vi "Fetch Waveform Measurement In Memory.vi"(6 "Measurement Number (0: Measurement 1)":i32(ring) items=["Measurement 1", "Measurement 2", "Measurement 3", "Measurement 4"], 7 "Destination Channel (1: Channel 2)":u16(ring)=1 items=["Channel 1", "Channel 2", "Channel 3", "Channel 4", "Math", "D0", "D1", "D2", "D3", "D4", "D5", "D6", "D7", "D8", "D9", "D10", "D11", "D12", "D13", "D14", "D15", "Reference 1", "Reference 2", "Reference 3", "Reference 4", "Amplitude", "Frequency", "Phase"], 8 "error in (no error)":errorcluster, 9 "Measurement Function (21: Period)":i32(ring)=21 items=["Amplitude", "Area", "Burst Width", "Cycle Area", "Voltage Mean (cycle)", "Voltage RMS (cycle)", "Delay", "Fall Time", "Frequency", "Voltage High", "Voltage Low", "Voltage Max", "Voltage Mean", "Voltage Min", "Negative Duty Cycle", "Negative Edges Count", "Negative Overshoot", "Negative Pulses Count", "Negative Pulse Width", "Positive Duty Cycle", "Positive Edges Count", "Period", "Phase", "Vpp", "Positive Overshoot", "Positive Pulses Count", "Positive Pulse Width", "Rise Time", "Voltage RMS"], 10 "Channel (0: Channel 1)":u16(ring) items=["Channel 1", "Channel 2", "Channel 3", "Channel 4", "Math", "D0", "D1", "D2", "D3", "D4", "D5", "D6", "D7", "D8", "D9", "D10", "D11", "D12", "D13", "D14", "D15", "Reference 1", "Reference 2", "Reference 3", "Reference 4", "Amplitude", "Frequency", "Phase"], 11 "VISA resource name":refnum<visa-resource-name>) -> (0 "error out":errorcluster, 2 "Measurement Value":dbl, 3 "VISA resource name out":refnum<visa-resource-name>)   [LabVIEW 2009, in "Tektronix DPO MSO 2000 4000 Series.lvlib"]
doc: "This VI fetches the displayed measurement value which is specified by the <B>Measurement Number</B>. \n\nFirstly, initiates an acquisition on the channel that you specify in the <B>Channel</B> control. After the acquisition completes, the Fetch Displayed Waveform Measurement VI performs displayed waveform measurement on the channel you specify and returns a measurement value. You can specify a measurement type, such as rise time, frequency, and voltage peak-to-peak, with this VI. Use the Fetch Displayed Waveform Measurement VI separately for any other waveform measurement on a channel without initiating another acquisition.\n\n<B>Notes:</B>\n\nThe <B>Fetch Waveform Measurement</B> VI returns the immediate measurement (which is what is typically done) while this VI returns the specified displayed measurement."
uses:
  <instrlib>/Tektronix DPO MSO 2000 4000 Series/Tektronix DPO MSO 2000 4000 Series.lvlib
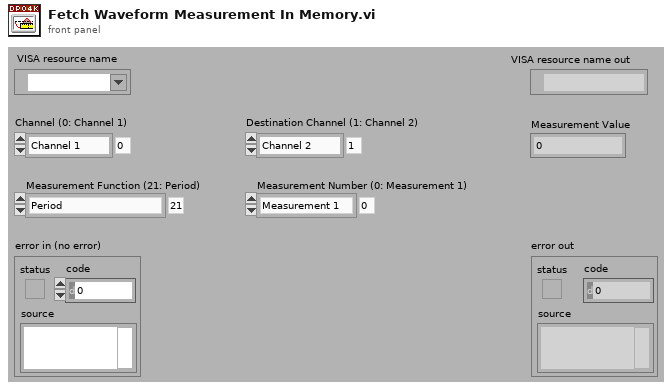
[diagram p1: front panel]
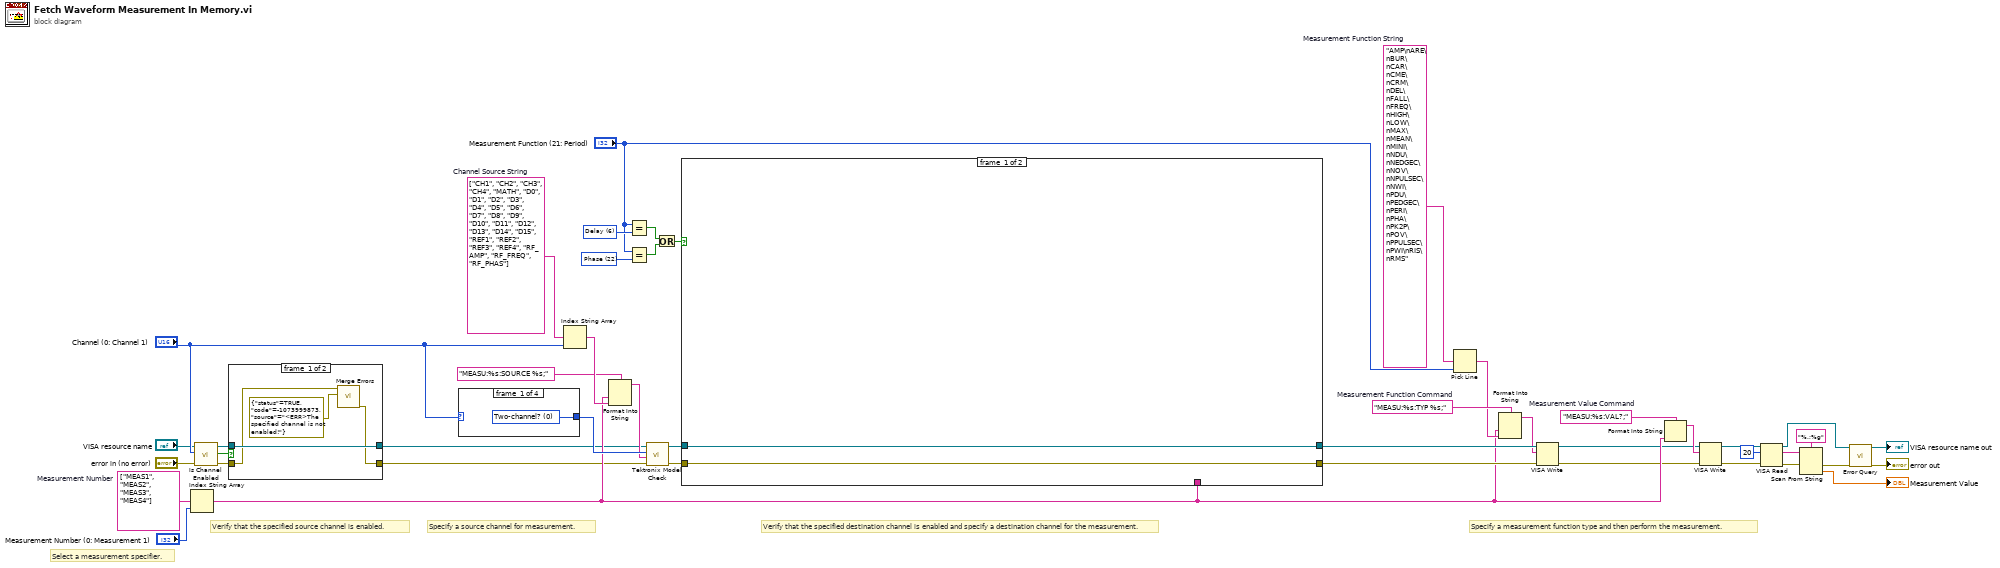
[diagram p0: block diagram]
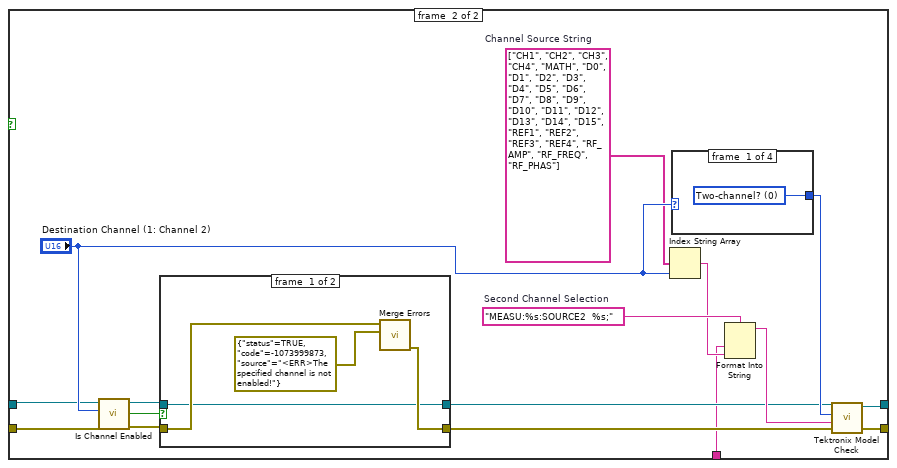
[diagram p2: hidden frame]
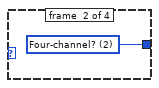
[diagram p3: hidden frame]
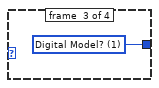
[diagram p4: hidden frame]
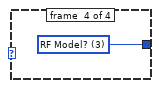
[diagram p5: hidden frame]
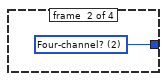
[diagram p7: hidden frame]
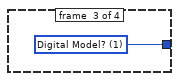
[diagram p8: hidden frame]
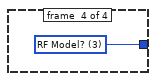
[diagram p9: hidden frame]
diagram:
  w11 = string[] ["MEAS1", "MEAS2", "MEAS3", "MEAS4"]  # Measurement Number
  w13 = "MEASU:%s:VAL?;"  # Measurement Value Command
  w28 = 22 items=["Amplitude", "Area", "Burst Width", "Cycle Area", "Voltage Mean (cycle)", "Voltage RMS (cycle)", "Delay", "Fall Time", "Frequency", "Voltage High", "Voltage Low", "Voltage Max", "Voltage Mean", "Voltage Min", "Negative Duty Cycle", "Negative Edges Count", "Negative Overshoot", "Negative Pulses Count", "Negative Pulse Width", "Positive Duty Cycle", "Positive Edges Count", "Period", "Phase", "Vpp", "Positive Overshoot", "Positive Pulses Count", "Positive Pulse Width", "Rise Time", "Voltage RMS"] ("Measurement Function (21: Period)")
  w29 = 6 items=["Amplitude", "Area", "Burst Width", "Cycle Area", "Voltage Mean (cycle)", "Voltage RMS (cycle)", "Delay", "Fall Time", "Frequency", "Voltage High", "Voltage Low", "Voltage Max", "Voltage Mean", "Voltage Min", "Negative Duty Cycle", "Negative Edges Count", "Negative Overshoot", "Negative Pulses Count", "Negative Pulse Width", "Positive Duty Cycle", "Positive Edges Count", "Period", "Phase", "Vpp", "Positive Overshoot", "Positive Pulses Count", "Positive Pulse Width", "Rise Time", "Voltage RMS"] ("Measurement Function (21: Period)")
  w37 = string[] ["CH1", "CH2", "CH3", "CH4", "MATH", "D0", "D1", "D2", "D3", "D4", "D5", "D6", "D7", "D8", "D9", "D10", "D11", "D12", "D13", "D14", "D15", "REF1", "REF2", "REF3", "REF4", "RF_AMP", "RF_FREQ", "RF_PHAS"]  # Channel Source String
  w44 = "MEASU:%s:TYP %s;"  # Measurement Function Command
  w45 = "AMP\nARE\nBUR\nCAR\nCME\nCRM\nDEL\nFALL\nFREQ\nHIGH\nLOW\nMAX\nMEAN\nMINI\nNDU\nNEDGEC\nNOV\nNPULSEC\nNWI\nPDU\nPEDGEC\nPERI\nPHA\nPK2P\nPOV\nPPULSEC\nPWI\nRIS\nRMS"  # Measurement Function String
  # "Select a measurement specifier."
  # "Specify a measurement function type and then perform the measurement."
  # "Specify a source channel for measurement."
  # "Verify that the specified destination channel is enabled and specify a destination channel for the measurement."
  # "Verify that the specified source channel is enabled."
  n1 = Index String Array(1:"Measurement Number (0: Measurement 1)", 2:w11) -> (0:w9:string)  [unwired: 1 in]
  n2 = call <instrlib>:"Is Channel Enabled.vi"("error in (no error)"="error in (no error)", "Channel (0: Channel 1)"="Channel (0: Channel 1)", "VISA resource name"="VISA resource name") -> ("error out"=w40:errorcluster, "Enabled"=w41:bool, "VISA resource name out"=w39:refnum<visa-resource-name>)  [unwired: 6 in]
  n3 = case shown="False" w41 {
    tunnel: w40 -> [w47 w50]
    tunnel: w39 -> [w48 w51]
    tunnel: [w48 w51] -> w4
    tunnel: [w46 w50] -> w3
    frame #0 {
      n4 = call <vilib>:"Merge Errors.vi"("error in 2 (no error)"=errorcluster {"status"=TRUE, "code"=-1073999873, "source"="<ERR>The specified channel is not enabled!"} ("error out"), "error in 1 (no error)"=w47) -> ("error out"=w46:errorcluster)  [unwired: 5 in]
    }
    frame #1 {
    }
  }
  n5 = case shown="0, 1, 4, 21..24, Default" "Channel (0: Channel 1)" {
    tunnel: [w52 w53 w54 w55] -> w38
    frame #0 {
      w52 = u16 0 items=["Two-channel?", "Digital Model?", "Four-channel?", "RF Model?"] ("Oscilloscope Model Tests (3: RF Model?)")
    }
    frame #1 {
      w53 = u16 2 items=["Two-channel?", "Digital Model?", "Four-channel?", "RF Model?"] ("Oscilloscope Model Tests (3: RF Model?)")
    }
    frame #2 {
      w54 = u16 1 items=["Two-channel?", "Digital Model?", "Four-channel?", "RF Model?"] ("Oscilloscope Model Tests (3: RF Model?)")
    }
    frame #3 {
      w55 = u16 3 items=["Two-channel?", "Digital Model?", "Four-channel?", "RF Model?"] ("Oscilloscope Model Tests (3: RF Model?)")
    }
  }
  n6 = Index String Array(1:"Channel (0: Channel 1)", 2:w37) -> (0:w35:string)  [unwired: 1 in]
  n7 = Format Into String(format string="MEASU:%s:SOURCE %s;", w9, w35) -> (resulting string=w33:string)  [unwired: 2 in, 1 out]
  n8 = Equal?(x="Measurement Function (21: Period)", y=w29) -> (x = y?=w30:bool)
  n9 = Equal?(x="Measurement Function (21: Period)", y=w28) -> (x = y?=w31:bool)
  n10 = call <instrlib>:"Tektronix Model Check.vi"("error in (no error)"=w3, "Command String"=w33, "Oscilloscope Model Tests (3: RF Model?)"=w38, "VISA resource name"=w4) -> ("error out"=w7:errorcluster, "VISA resource name out"=w8:refnum<visa-resource-name>)  [unwired: 6 in]
  n11 = Or(x=w30, y=w31) -> (x .or. y?=w27:bool)
  n12 = case shown="False" w27 {
    tunnel: w8 -> [w57 w64]
    tunnel: w7 -> [w56 w63]
    tunnel: [w57 w62] -> w25
    tunnel: [w56 w61] -> w24
    tunnel: w9 -> [_ w58]
    frame #0 {
    }
    frame #1 {
      w68 = string[] ["CH1", "CH2", "CH3", "CH4", "MATH", "D0", "D1", "D2", "D3", "D4", "D5", "D6", "D7", "D8", "D9", "D10", "D11", "D12", "D13", "D14", "D15", "REF1", "REF2", "REF3", "REF4", "RF_AMP", "RF_FREQ", "RF_PHAS"]  # Channel Source String
      w60 = "MEASU:%s:SOURCE2  %s;"  # Second Channel Selection
      n13 = call <instrlib>:"Is Channel Enabled.vi"("error in (no error)"=w63, "Channel (0: Channel 1)"="Destination Channel (1: Channel 2)", "VISA resource name"=w64) -> ("error out"=w67:errorcluster, "Enabled"=w65:bool, "VISA resource name out"=w66:refnum<visa-resource-name>)  [unwired: 6 in]
      n14 = case shown="True" w65 {
        tunnel: w66 -> [w78 w83]
        tunnel: w67 -> [w80 w82]
        tunnel: [w78 w83] -> w69
        tunnel: [w79 w82] -> w70
        frame #0 {
          n15 = call <vilib>:"Merge Errors.vi"("error in 2 (no error)"=errorcluster {"status"=TRUE, "code"=-1073999873, "source"="<ERR>The specified channel is not enabled!"} ("error out"), "error in 1 (no error)"=w80) -> ("error out"=w79:errorcluster)  [unwired: 5 in]
        }
        frame #1 {
        }
      }
      n16 = Index String Array(1:"Destination Channel (1: Channel 2)", 2:w68) -> (0:w59:string)  [unwired: 1 in]
      n17 = case shown="0, 1, 4, 21..24, Default" "Destination Channel (1: Channel 2)" {
        tunnel: [w74 w75 w76 w77] -> w73
        frame #0 {
          w74 = u16 0 items=["Two-channel?", "Digital Model?", "Four-channel?", "RF Model?"] ("Oscilloscope Model Tests (3: RF Model?)")
        }
        frame #1 {
          w75 = u16 2 items=["Two-channel?", "Digital Model?", "Four-channel?", "RF Model?"] ("Oscilloscope Model Tests (3: RF Model?)")
        }
        frame #2 {
          w76 = u16 1 items=["Two-channel?", "Digital Model?", "Four-channel?", "RF Model?"] ("Oscilloscope Model Tests (3: RF Model?)")
        }
        frame #3 {
          w77 = u16 3 items=["Two-channel?", "Digital Model?", "Four-channel?", "RF Model?"] ("Oscilloscope Model Tests (3: RF Model?)")
        }
      }
      n18 = Format Into String(format string=w60, w58, w59) -> (resulting string=w71:string)  [unwired: 2 in, 1 out]
      n19 = call <instrlib>:"Tektronix Model Check.vi"("error in (no error)"=w70, "Command String"=w71, "Oscilloscope Model Tests (3: RF Model?)"=w73, "VISA resource name"=w69) -> ("error out"=w61:errorcluster, "VISA resource name out"=w62:refnum<visa-resource-name>)  [unwired: 6 in]
    }
  }
  n20 = Pick Line(multi-line string=w45, line index="Measurement Function (21: Period)") -> (output string=w32:string)  [unwired: 1 in]
  n21 = Format Into String(format string=w44, w9, w32) -> (resulting string=w23:string)  [unwired: 2 in, 1 out]
  n22 = VISA Write(VISA resource name=w25, write buffer=w23, error in (no error)=w24) -> (VISA resource name out=w6:refnum<visa-resource-name>, error out=w5:errorcluster)  [unwired: 1 out]
  n23 = Format Into String(format string=w13, w9) -> (resulting string=w12:string)  [unwired: 2 in, 1 out]
  n24 = VISA Write(VISA resource name=w6, write buffer=w12, error in (no error)=w5) -> (VISA resource name out=w21:refnum<visa-resource-name>, error out=w20:errorcluster)  [unwired: 1 out]
  n25 = VISA Read(VISA resource name=w21, byte count=u32 20, error in (no error)=w20) -> (VISA resource name out=w17:refnum<visa-resource-name>, read buffer=w16:string, error out=w18:errorcluster)  [unwired: 1 out]
  n26 = Scan From String(format string="%.;%g", input string=w16, error in=w18) -> (error out=w15:errorcluster, output 1=→"Measurement Value":dbl)  [unwired: 2 in, 2 out]
  n27 = call <instrlib>:"Error Query.vi"("error in (no error)"=w15, "VISA resource name"=w17) -> ("error out"=→"error out":errorcluster, "VISA resource name out"=→"VISA resource name out":refnum<visa-resource-name>)  [unwired: 6 in, 2 out]
